vi "get_config_cluster.vi"(8 "error in (no error)":errorcluster, 11 "TrajectoryRK110916Throughput in":refnum<class "TrajectoryRK110916Throughput.lvclass">) -> (0 "error out":errorcluster, 2 "config cluster (variant)":variant, 3 "TrajectoryRK110916Throughput out":refnum<class "TrajectoryRK110916Throughput.lvclass">)   [LabVIEW 2010, in "TrajectoryRK110916Throughput.lvclass"]
uses:
  TrajectoryRK110916Throughput.lvclass
  TrajectoryRK110916Throughput.lvclass/TrajectoryRK110916Throughput.ctl
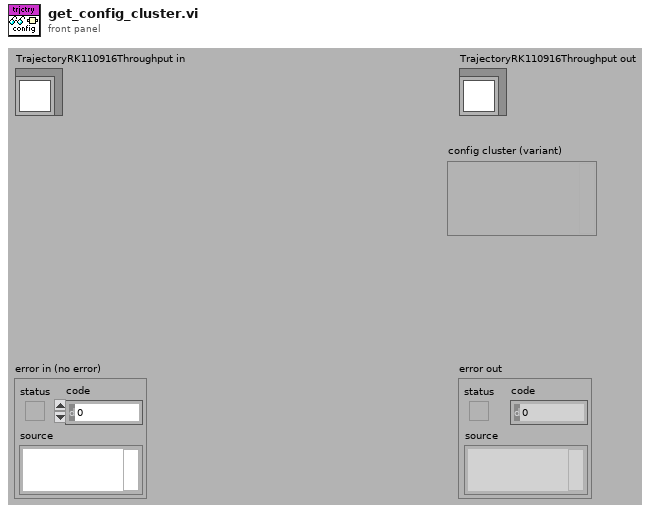
[diagram p1: front panel]
types:
  T1 = typedef "TrajectoryRK110916Throughput.lvclass/config_data_cluster.ctl" = cluster{"FGPA clockspeed":dbl}
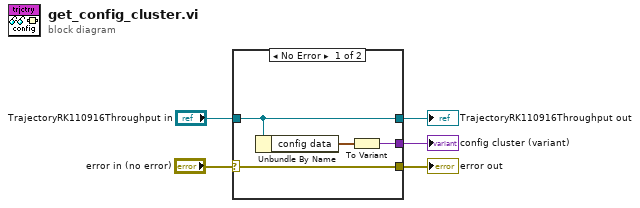
[diagram p0: block diagram]
diagram:
  n1 = case shown="No Error" "error in (no error)" {
    selector: "error in (no error)" -> [w9 w11]
    tunnel: [w9 w11] -> w4
    tunnel: "TrajectoryRK110916Throughput in" -> [w8 w10]
    tunnel: [w8 w10] -> w2
    tunnel: [w6 _] -> w1
    frame No Error {
      n2 = Unbundle By Name(w8) -> ("config data"=w7:T1)
      n3 = To Variant(anything=w7) -> (Variant=w6:variant)
    }
    frame Error {
    }
  }
  "error out" <- w4
  "TrajectoryRK110916Throughput out" <- w2
  "config cluster (variant)" <- w1
